vi "pos_front2back.vi"(8 "error in (no error)":errorcluster, 10 "pos frontend":dbl, 11 "Motor in":refnum<class "Motor.lvclass">) -> (0 "error out":errorcluster, 2 "pos backend":dbl, 3 "Motor out":refnum<class "Motor.lvclass">)   [LabVIEW 2016, in "Hardware.lvlib" / "Motor.lvlib" / "Motor.lvclass"]
uses:
  <userlib>/Common Components/Hardware/Motor/Motor/Motor.lvclass
  <userlib>/Common Components/Hardware/Motor/Motor/Motor.lvclass/Motor.ctl
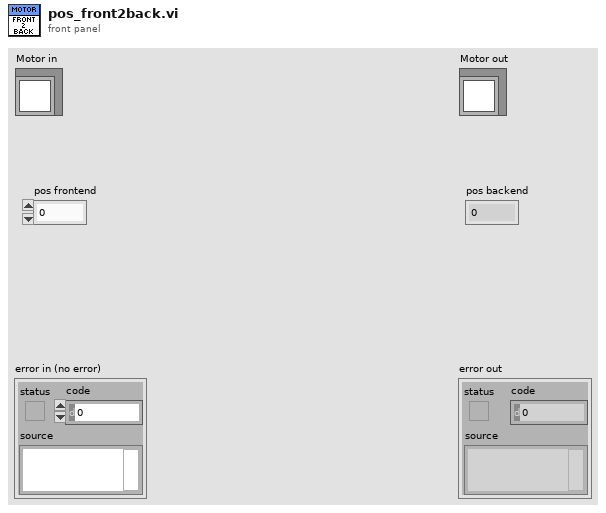
[diagram p1: front panel]
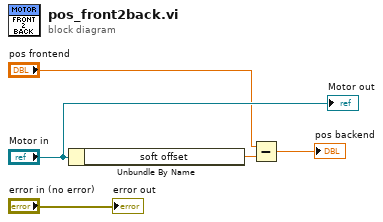
[diagram p0: block diagram]
diagram:
  n1 = Unbundle By Name("Motor in") -> ("soft offset"=w1:dbl)
  n2 = Subtract(x="pos frontend", y=w1) -> (x-y=→"pos backend":dbl)
  "error out" <- "error in (no error)"
  "Motor out" <- "Motor in"
